vi "Read User Events.vi"(8 "error in (no error)":errorcluster, 11 "EMS Generic in":refnum<class "EMS Generic.lvclass">) -> (0 "error out":errorcluster, 2 "user events":T1, 3 "EMS Generic out":refnum<class "EMS Generic.lvclass">)   [LabVIEW 2018, in "EMS Generic Actor.lvlib" / "EMS Generic.lvclass"]
uses:
  EMS Generic.lvclass
  Controls/EMS Generic User Events.ctl
  EMS Generic.lvclass/EMS Generic.ctl
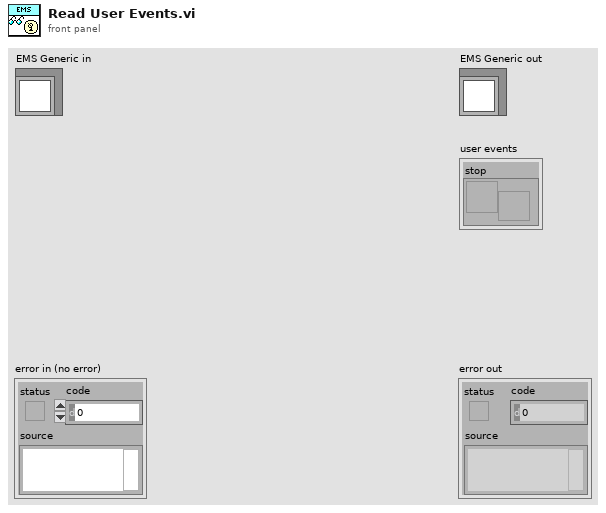
[diagram p1: front panel]
types:
  T1 = typedef "EMS Generic Actor.lvlib/EMS Generic.lvclass/EMS Generic User Events.ctl" = cluster{"stop":refnum<user-event>}
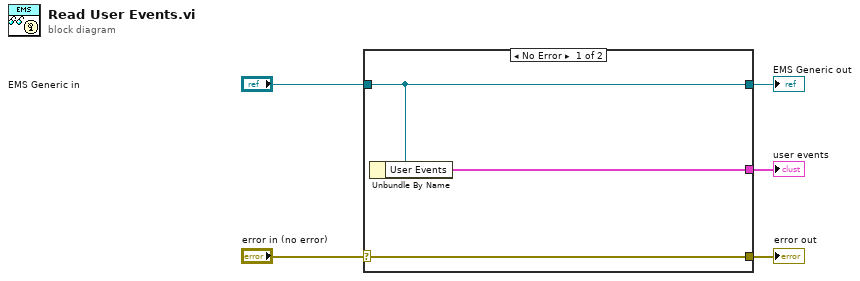
[diagram p0: block diagram]
diagram:
  n1 = case shown="No Error" "error in (no error)" {
    selector: "error in (no error)" -> [w8 w9]
    tunnel: [w8 w9] -> w4
    tunnel: [w7 w10] -> w2
    tunnel: "EMS Generic in" -> [w7 w10]
    tunnel: [w6 _] -> w1
    frame No Error {
      n2 = Unbundle By Name(w7) -> ("User Events"=w6:T1)
    }
    frame Error {
    }
  }
  "error out" <- w4
  "EMS Generic out" <- w2
  "user events" <- w1
